vi "Delta range (seq) (SubVI).vi"(10 "字符串":string, 11 "队列输入":refnum<queue>) -> (0 "错误输出":errorcluster)   [LabVIEW 2019, in "Take Seq.lvlib"]
uses:
  Take Seq.lvlib
  config.ctl
  Instrument.ctl
  lib/QDInstrument.dll
  <vilib>/NI/Modbus Library/API/Master/Modbus Master.lvclass
  lib/Keithley 622x/Configure/2182 -A/Low Level/Typedefs/KE2182 -- Voltage Ranges.ctl
  lib/Keithley 622x/Keithley 622x.lvlib
panel:
  # "(真是通道1，假是通道2)"
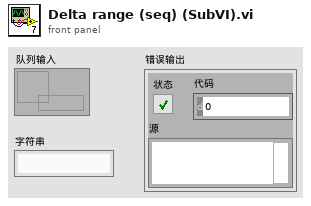
[diagram p1: front panel]
types:
  T1 = typedef "config.ctl" = cluster{"initialize":string, "6221":cluster{"6221 Resource":refnum<visa-resource-name>, "Delta status":bool}, "7001":cluster{"Ch":bool}, "SR830+6221":cluster{"source":u16, "阻抗":dbl, "量程入 4":i32, "量程入 3":i32, "量程入 2":i32, "量程入 1":i32, "电流":dbl, "SR830 2":bool, "SR830 3":bool, "SR830 4":bool, "SR830 1":bool, "VISA 1":refnum<visa-resource-name>, "VISA 2":refnum<visa-resource-name>, "VISA 3":refnum<visa-resource-name>, "VISA 4":refnum<visa-resource-name>, "量程":enum16{"量程每次测量会判定", "量程不变为设定值"}}, "2400":cluster{"2400":bool, "VISA":refnum<visa-resource-name>}, "ch":cluster{"ch str":string, "ch1":bool, "ch2":bool, "布尔":bool}, "error":bool, "数据文件路径":path, "log":cluster{"log路径":path, "log interval":dbl}, "Instrument":T2}
  T2 = typedef "Instrument.ctl" = cluster{"335 Resource":refnum<visa-resource-name>, "Input (0:A)":u16, "Instrument Type":i32, "quantum design":refnum<k24>, "Heater Output (1:1)":u16, "335state":refnum<vi>, "semaphore":T3, "TCP master instance":refnum<class "Modbus Master.lvclass">}
  T3 = typedef "Semaphore RefNum" = refnum<k1>
  T4 = typedef "Keithley 622x.lvlib/KE2182 -- Voltage Ranges.ctl" = enum16{"10mV", "100mV", "1V", "10V", "100V"}
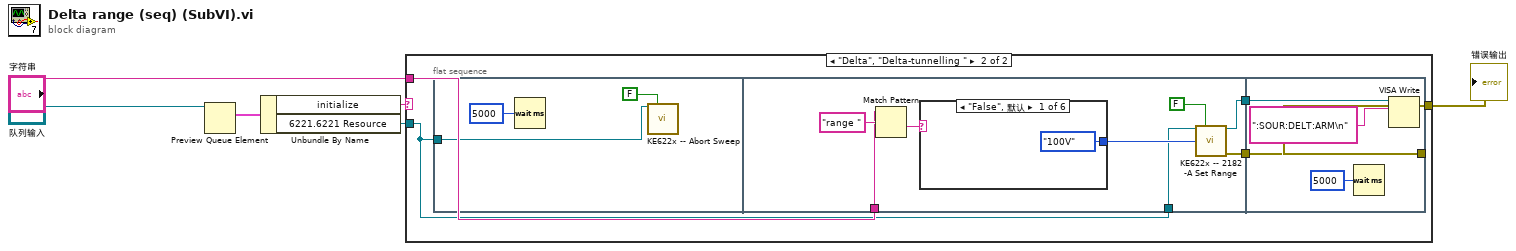
[diagram p0: block diagram]
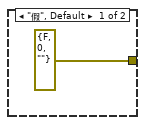
[diagram p2: hidden frame]
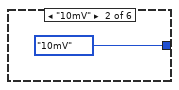
[diagram p3: hidden frame]
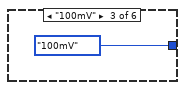
[diagram p4: hidden frame]
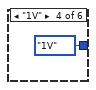
[diagram p5: hidden frame]
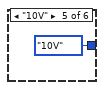
[diagram p6: hidden frame]
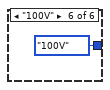
[diagram p7: hidden frame]
diagram:
  n1 = Preview Queue Element(queue="队列输入") -> (element=w2:T1)  [unwired: 2 in, 3 out]
  n2 = Unbundle By Name(w2) -> ("initialize"=w3:string, "6221.6221 Resource"=w6:refnum<visa-resource-name>)
  n3 = case shown="\"Delta\", \"Delta-tunnelling \"" w3 {
    tunnel: "字符串" -> [_ w12]
    tunnel: w6 -> [_ w10]
    tunnel: [errorcluster {"status"=FALSE, "code"=0, "source"=""} ("error out") w11] -> w5
    frame "假", Default {
    }
    frame "Delta", "Delta-tunnelling " {
      n4 = flat-sequence {
        tunnel: w10 -> [w14]
        tunnel: w12 -> [w21]
        tunnel: w10 -> [w19]
        tunnel: [w17] -> w9
        tunnel: [w16] -> w8
        tunnel: [w33] -> w11
        tunnel: w9 -> [w33]
        tunnel: w8 -> [w32]
        frame #0 {
          n5 = Wait (ms)(milliseconds to wait=u32 5000) -> ()  [unwired: 1 out]
          n6 = call "KE622x -- Abort Sweep.vi"("Resource In"=w14, "Check For SCPI Errors? (T)"=FALSE) -> ()  [unwired: 12 in, 2 out]
        }
        frame #1 {
          n7 = Match Pattern(string=w21, regular expression="range ") -> (after substring=w22:string)  [unwired: 1 in, 3 out]
          n8 = case shown="\"False\", 默认" w22 {
            tunnel: [KE2182_--_Voltage_Ranges."100V" ("Man / Selected\nRange") KE2182_--_Voltage_Ranges."10mV" ("Man / Selected\nRange") KE2182_--_Voltage_Ranges."100mV" ("Man / Selected\nRange") KE2182_--_Voltage_Ranges."1V" ("Man / Selected\nRange") KE2182_--_Voltage_Ranges."10V" ("Man / Selected\nRange") KE2182_--_Voltage_Ranges."100V" ("Man / Selected\nRange")] -> w20
            frame "False", Default {
            }
            frame "10mV" {
            }
            frame "100mV" {
            }
            frame "1V" {
            }
            frame "10V" {
            }
            frame "100V" {
            }
          }
          n9 = call "KE622x -- 2182 -A Set Range.vi"("622x Resource In"=w19, "Check For SCPI Errors? (T)"=FALSE, "2182/2182A Range"=w20) -> ("622x Resource Out (dupl)"=w16:refnum<visa-resource-name>, "error out"=w17:errorcluster)  [unwired: 11 in]
        }
        frame #2 {
          n10 = Wait (ms)(milliseconds to wait=u32 5000 ("等待时间（毫秒）")) -> ()  [unwired: 1 out]
          n11 = VISA Write(VISA resource name=w32, write buffer=":SOUR:DELT:ARM\n" ("format string")) -> ()  [unwired: 1 in, 3 out]
        }
      }
    }
  }
  "错误输出" <- w5
